vi "S1Ouputs.vi"(8 "error in":errorcluster, 11 "SIOutputs":T1) -> (0 "error out":errorcluster)   [LabVIEW 2018, in "IO.lvclass"]
uses:
  IO.lvclass
  S1/Public Controls/Outputs.ctl
  Queue/Queue Data.ctl
  Queue/State.ctl
  5d0634fd-1950-45e8-a22d-fdfd28c003d0.vi
  S1/S1.lvclass
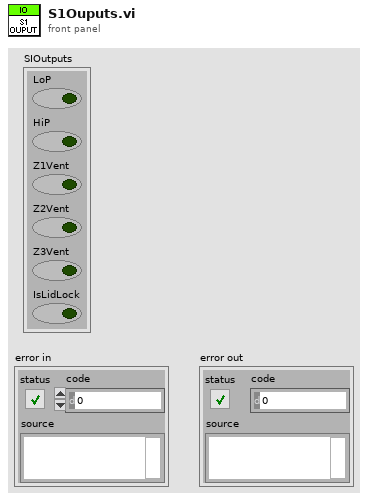
[diagram p1: front panel]
types:
  T1 = typedef "S1.lvclass/Outputs.ctl" = cluster{"LoP":bool, "HiP":bool, "Z1Vent":bool, "Z2Vent":bool, "Z3Vent":bool, "IsLidLock":bool}
  T2 = typedef "IO.lvclass/Queue Data.ctl" = cluster{"State":T3, "Data":variant}
  T3 = typedef "IO.lvclass/State.ctl" = enum16{"Initialize", "GlobalConfig", "ESTOP", "Abort", "S1Ouputs", "S2Outputs", "S3Ouputs", "S4Outputs", "S5Outputs", "S6Outputs", "Read", "Error", "Exit"}
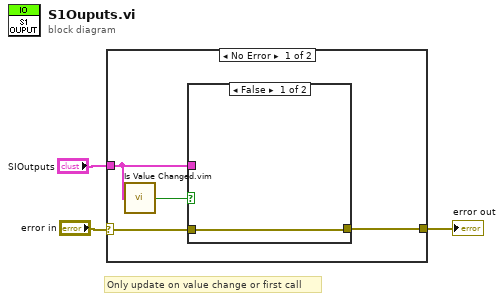
[diagram p0: block diagram]
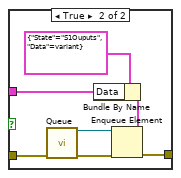
[diagram p2: hidden frame]
diagram:
  # "Only update on value change or first call"
  n1 = case shown="No Error" "error in" {
    selector: "error in" -> [w7 w16]
    tunnel: [w6 w16] -> w3
    tunnel: "SIOutputs" -> [w5 _]
    frame No Error {
      n2 = call "Is Value Changed.vim"("value"=w5) -> ("changed or first call?"=w4:bool)
      n3 = case shown="False" w4 {
        tunnel: w7 -> [w8 w15]
        tunnel: [w8 w14] -> w6
        tunnel: w5 -> [_ w9]
        frame False {
        }
        frame True {
          n4 = call "Queue.vi"("error in"=w15) -> ("error out"=w13:errorcluster, "queue out"=w12:refnum<queue>)  [unwired: 9 in]
          n5 = Bundle By Name(cluster=T2 {"State"=enum."S1Ouputs", "Data"=variant} ("element"), "Data"=w9) -> (w10:T2)
          n6 = Enqueue Element(queue=w12, element=w10, error in (no error)=w13) -> (error out=w14:errorcluster)  [unwired: 1 in, 2 out]
        }
      }
    }
    frame Error {
    }
  }
  "error out" <- w3
